vi "Inform Result File Path.vi"(0 "Result File Path":path, 5 "DUT Site":i32, 7 "DUT Pin":string, 11 "error in":errorcluster) -> (15 "error out":errorcluster)   [LabVIEW 2023, in "RFFixtureCharact.RFPM.lvlib" / "Charact Result Accessor.lvclass"]
uses:
  Charact Result Accessor.lvclass
  Common/RFCalAndFixtureCharact.Common.lvlib
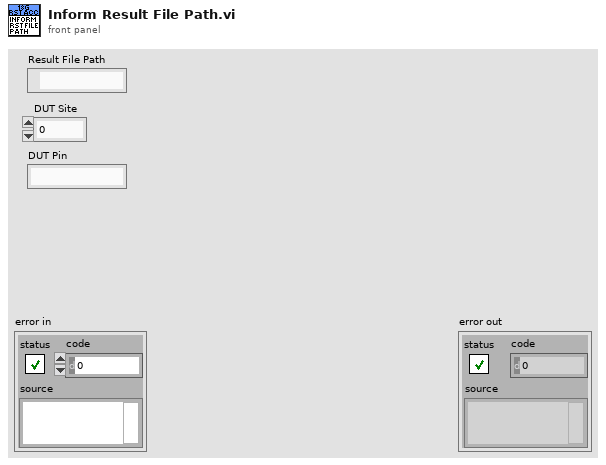
[diagram p1: front panel]
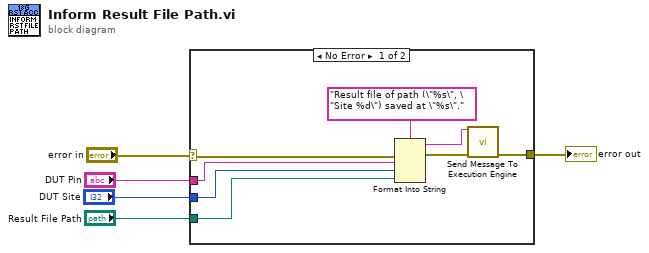
[diagram p0: block diagram]
diagram:
  n1 = case shown="No Error" "error in" {
    selector: "error in" -> [w9 w14]
    tunnel: [w11 w14] -> w4
    tunnel: "Result File Path" -> [w8 _]
    tunnel: "DUT Pin" -> [w7 _]
    tunnel: "DUT Site" -> [w6 _]
    frame No Error {
      n2 = Format Into String(format string="Result file of path (\"%s\", \"Site %d\") saved at \"%s\".", error in=w9, w7, w6, w8) -> (resulting string=w10:string, error out=w13:errorcluster)  [unwired: 1 in]
      n3 = call "Send Message To Execution Engine.vi"("Message"=w10, "error in (no error)"=w13) -> ("error out"=w11:errorcluster)  [unwired: 13 in]
    }
    frame Error {
    }
  }
  "error out" <- w4
